vi "Setup.vi"(8 "error in (no error)":errorcluster, 11 "EventFile in":refnum<class "EventFile.lvclass">) -> (0 "error out":errorcluster, 3 "EventFile out":refnum<class "EventFile.lvclass">)   [LabVIEW 2016, in "Event Logging.lvlib" / "EventFile.lvclass"]
uses:
  EventFile.lvclass
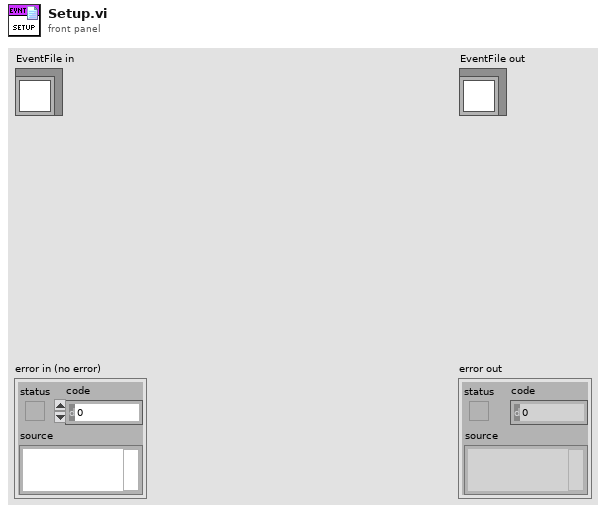
[diagram p1: front panel]
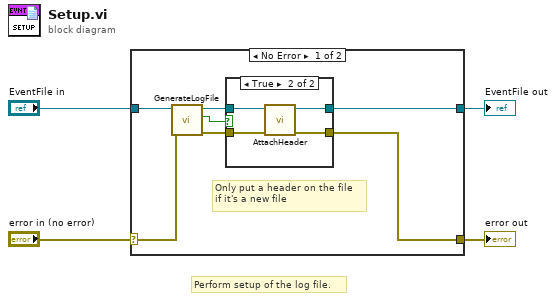
[diagram p0: block diagram]
diagram:
  # "Perform setup of the log file."
  n1 = case shown="No Error" "error in (no error)" {
    selector: "error in (no error)" -> [w10 w19]
    tunnel: [w5 w19] -> w3
    tunnel: [w7 w18] -> w1
    tunnel: "EventFile in" -> [w11 w18]
    frame No Error {
      # "Only put a header on the file\nif it's a new file"
      n2 = call-dynamic "GenerateLogFile.vi"("error in (no error)"=w10, "EventFile in"=w11) -> ("error out"=w6:errorcluster, "newFile?"=w9:bool, "EventFile out"=w8:refnum<class "EventFile.lvclass">)  [unwired: 7 in]
      n3 = case shown="True" w9 {
        tunnel: w8 -> [w13 w17]
        tunnel: [w13 w16] -> w7
        tunnel: w6 -> [w12 w15]
        tunnel: [w12 w14] -> w5
        frame False {
        }
        frame True {
          n4 = call-dynamic "AttachHeader.vi"("error in (no error)"=w15, "EventFile in"=w17) -> ("error out"=w14:errorcluster, "EventFile out"=w16:refnum<class "EventFile.lvclass">)  [unwired: 8 in]
        }
      }
    }
    frame Error {
    }
  }
  "error out" <- w3
  "EventFile out" <- w1
